vi "DT9816_Multiplexer.vi"(0 "Sample Freq (Hz)":dbl=1000.0, 1 "Samples Per Channel":u32=100, 2 "Sample Mode":enum16{"Finite Samples", "Continuous Samples"}(ring)=enum."Continuous Samples", 3 "Multiplexer cycle freq. (Hz)":dbl=200.0, 6 "Number Chan to Read":u32=6, 8 "Channel list (Ain5 for channel volts)":string="0:4, 5", 9 "Vmax":dbl=10.0, 10 "Board Name":string="DT9816(00)", 11 "Vmin":dbl=-10.0, 12 "N banks":i32=8, 13 "Clock Duty Cycle (%)":dbl=50.0) -> (14 "2D volts out":dbl[][](array[numeric]), 15 "Multiplexer bank no.":i32[](array[numeric])=[5, 4, 4, 4, 5, 5, 4, 4, 4, 5, 5, 4, 4, 4, 5, 5, 4, 4, 4, 5, 5, 4, 4, 4, 5, 5, 4, 4, 4, 5, 5, 4, 4, 4, 5, 5, 4, 4, 4, 5, 5, 4, 4, 4, 5, 5, 4, 4, 4, 5, 5, 4, 4, 4, 5, 5, 4, 4, 4, 5, 5, 4, 4, 4, 5, 5, 4, 4, 4, 5, 5, 4, 4, 4, 5, 5, 4, 4, 4, 5, 5, 4, 4, 4, 5, 5, 4, 4, 4, 5, 5, 4, 4, 4, 5, 5, 4, 4, 4, 5], 17 "Actual Sample Freq":dbl, 18 "Data acq. final error":errorcluster, 19 "Clock error":errorcluster)   [LabVIEW 2013]
uses:
  <userlib>/LV-Link3/PolySubVIs/DtCreateCtrRateChan.vi
  <userlib>/LV-Link3/PolySubVIs/DtOLStartNormal.vi
  <userlib>/LV-Link3/PolySubVIs/DtCreateAinChan.vi
  <userlib>/LV-Link3/PolySubVIs/DtOLTimingSetInput.vi
  <userlib>/LV-Link3/PolySubVIs/DtOLReadMultiple2D.vi
panel:
  in  "V_DACmax":dbl=10.0
  # "N.B. Digital IO must be LAST on the channel list"
  # "Clock is output on CTR0 (pin17)"
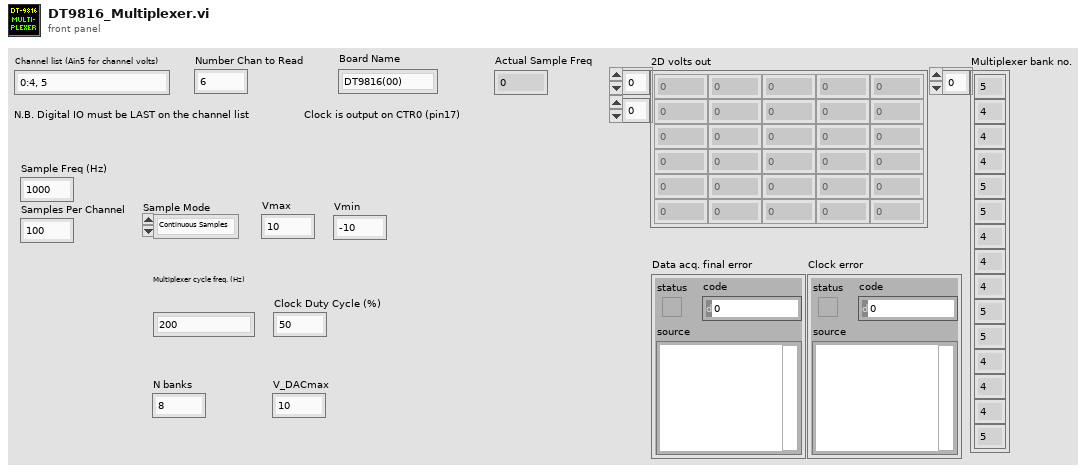
[diagram p1: front panel]
types:
  T1 = enum32{"Internal Clock", "External Clock", "No Timing"}
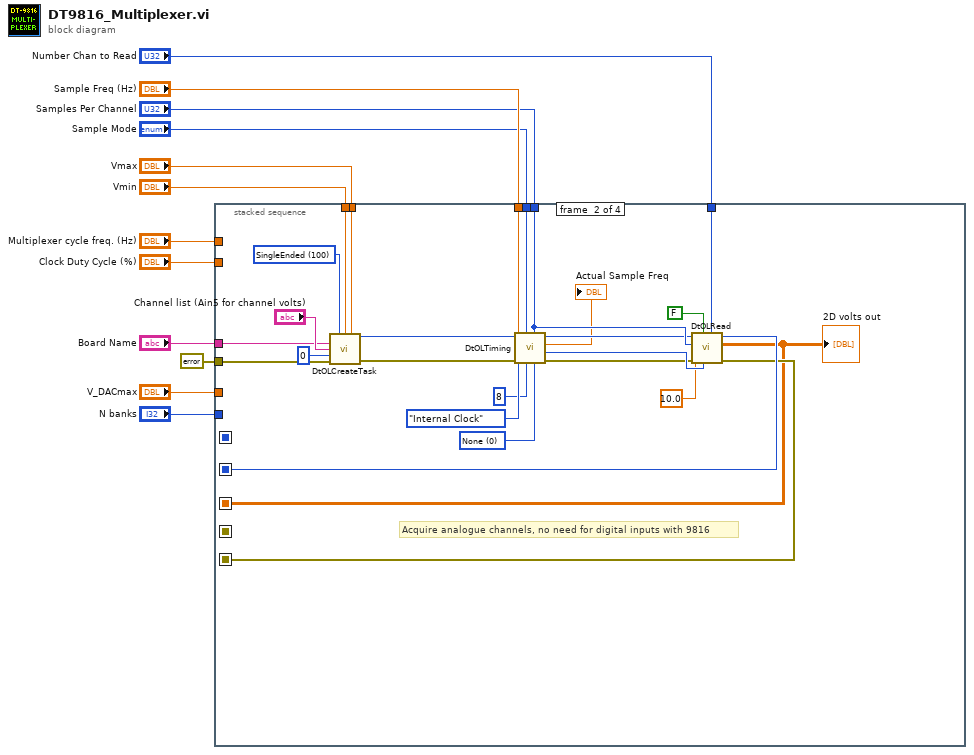
[diagram p0: block diagram]
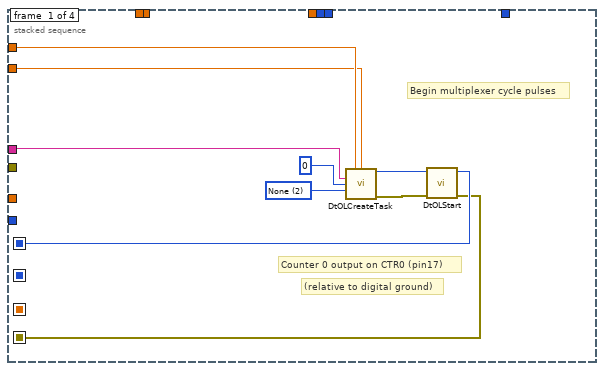
[diagram p2: hidden frame]
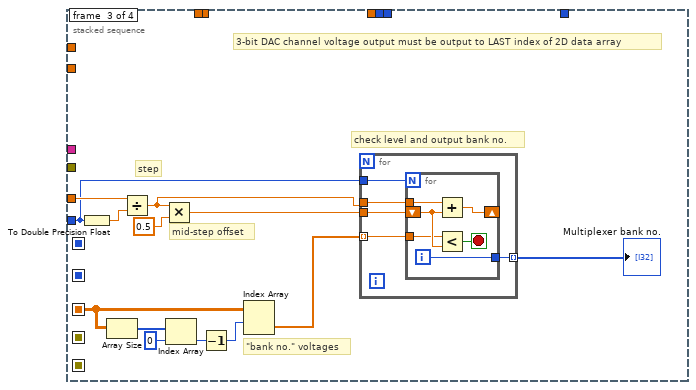
[diagram p3: hidden frame]
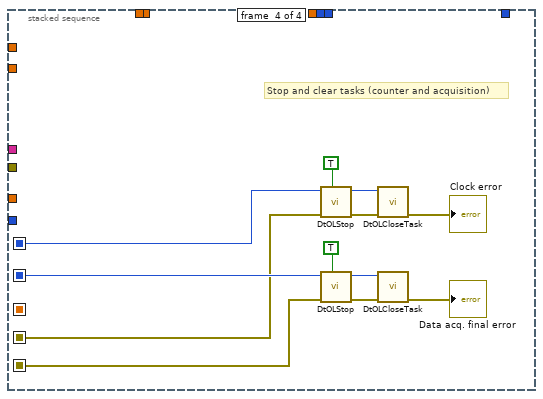
[diagram p4: hidden frame]
diagram:
  n1 = stacked-sequence {
    seq-local: [w15 _ _ _] -> [_ _ _ w72]
    seq-local: [_ w22 _ _] -> [_ _ w56 _]
    seq-local: [_ w25 _ _] -> [_ _ _ w77]
    seq-local: [_ w24 _ _] -> [_ _ _ w78]
    seq-local: [w14 _ _ _] -> [_ _ _ w71]
    tunnel: errorcluster {"status"=FALSE, "code"=0, "source"=""} ("error out") -> [_ w46 _ _]
    tunnel: "Sample Freq (Hz)" -> [_ w42 _ _]
    tunnel: "Sample Mode" -> [_ w39 _ _]
    tunnel: "Board Name" -> [w17 w36 _ _]
    tunnel: "Samples Per Channel" -> [_ w34 _ _]
    tunnel: "Number Chan to Read" -> [_ w31 _ _]
    tunnel: "Vmax" -> [_ w27 _ _]
    tunnel: "Vmin" -> [_ w26 _ _]
    tunnel: "Multiplexer cycle freq. (Hz)" -> [w16 _ _ _]
    tunnel: "Clock Duty Cycle (%)" -> [w13 _ _ _]
    tunnel: "V_DACmax" -> [_ _ w59 _]
    tunnel: "N banks" -> [_ _ w48 _]
    frame #0 {
      w20 = 2 items=["LowLevel", "HighLevel", "None"] ("Gate Type")
      # "Begin multiplexer cycle pulses"
      # "(relative to digital ground)"
      # "Counter 0 output on CTR0 (pin17)"
      n2 = call-poly <userlib>:"DtOLCreateTask.vi"("Requested\nFrequency (Hz)"=w16, "Duty Cycle"=w13, "Board Name"=w17, "Counter Num"=u32 0, "Gate Type"=w20) -> ("Task out"=w19:i32, "error out"=w18:errorcluster)  [unwired: 8 in, 1 out]
      n3 = call-poly <userlib>:"DtOLStart.vi"("error in (no error)"=w18, "Task in"=w19) -> ("error out"=w14:errorcluster, "Task out"=w15:i32)  [unwired: 8 in]
    }
    frame #1 {
      w37 = 0 items=["None", "Master", "Slave"] ("Sync Mode")
      w43 = 100 items=["SingleEnded"=100, "Differential"=101] ("Channel Type")
      # "Acquire analogue channels, no need for digital inputs with 9816"
      n4 = call-poly <userlib>:"DtOLCreateTask.vi"("Channel Type"=w43, "Range Min"=w26, "Range Max"=w27, "Board Name"=w36, "Channel"="Channel list (Ain5 for channel volts)", "Element"=u32 0, "error in (no error)"=w46) -> ("Task out"=w28:i32, "error out"=w40:errorcluster)  [unwired: 6 in, 1 out]
      n5 = call-poly <userlib>:"DtOLTiming.vi"("Sync Mode"=w37, "Samples Per Channel"=w34, "Num Buffers"=u32 8, "Sample Mode"=w39, "error in (no error)"=w40, "Timing"=T1."Internal Clock", "Sample Freq (Hz)"=w42, "Task in"=w28) -> ("error out"=w29:errorcluster, "Buffer Size"=w35:u32, "Actual Sample Freq"=→"Actual Sample Freq":dbl, "Task out"=w30:i32)
      n6 = call-poly <userlib>:"DtOLRead.vi"("Number Chan to Read"=w31, "Buffer size"=w35, "OnlyReadAvailable"=FALSE, "error in (no error)"=w29, "Timeout"=10.0, "Samples Per Channel"=w34, "Task in"=w30) -> ("error out"=w24:errorcluster, "2D Data out"=w22:dbl[][], "Task out"=w25:i32)  [unwired: 2 out]
      "2D volts out" <- w22
    }
    frame #2 {
      # "check level and output bank no."
      # "\"bank no.\" voltages"
      # "mid-step offset"
      # "step"
      # "3-bit DAC channel voltage output must be output to LAST index of 2D data array"
      n7 = To Double Precision Float(number=w48) -> (double precision float=w58:dbl)
      n8 = Array Size(array=w56) -> (size(s)=w54:i32[])
      n9 = Divide(x=w59, y=w58) -> (x/y=w49:dbl)
      n10 = Multiply(x=w49, y=0.5) -> (x*y=w51:dbl)
      n11 = Index Array(array=w54, index=0) -> (element=w53:i32)
      n12 = Decrement(x=w53) -> (x-1=w52:i32)
      n13 = Index Array(array=w56, index (row)=w52) -> (element=w50:dbl[])  [unwired: 1 in]
      n14 = for {
        tunnel: w50 -> [w62] mode=indexing
        tunnel: w51 -> [w64]
        tunnel: w49 -> [w63]
        tunnel: w48 -> [w61]
        tunnel: [w60] -> w47 mode=indexing
        n15 = for {
          N: w61 -> [_]
          shift-right: [w70] -> _
          shift-left: w64 -> [w68]
          tunnel: w63 -> [w69]
          tunnel: w62 -> [w67]
          tunnel: [w65] -> w60
          i -> [w65]
          stop <- w66 stop-if-true
          n16 = Add(x=w69, y=w68) -> (x+y=w70:dbl)
          n17 = Less?(x=w67, y=w68) -> (x < y?=w66:bool)
        }
      }
      "Multiplexer bank no." <- w47
    }
    frame #3 {
      # "Stop and clear tasks (counter and acquisition)"
      n18 = call <userlib>:"DtOLStop.vi"("Finish Buffer"=TRUE, "error in (no error)"=w71, "Task in"=w72) -> ("error out"=w75:errorcluster, "Task out"=w74:i32)  [unwired: 7 in]
      n19 = call <userlib>:"DtOLStop.vi"("Finish Buffer"=TRUE, "error in (no error)"=w78, "Task in"=w77) -> ("error out"=w80:errorcluster, "Task out"=w81:i32)  [unwired: 7 in]
      n20 = call <userlib>:"DtOLCloseTask.vi"("Error in"=w75, "Task in"=w74) -> ("Error Out"=→"Clock error":errorcluster)  [unwired: 9 in]
      n21 = call <userlib>:"DtOLCloseTask.vi"("Error in"=w80, "Task in"=w81) -> ("Error Out"=→"Data acq. final error":errorcluster)  [unwired: 9 in]
    }
  }
